vi "waveformTimeKeep.vi"(6 "DAQ Settings":T1={"RH/T Sensor VSS (V)"=5.048, "K0"=0.9054, "K1"=-2.995, "Offset"=0.0, "Gain"=1.0, "Samples/Channel/s"=1000.0, "Samples to Average"=100.0} {"Offset" step=0.01 format="%_3f"; "K1" format="%#_13g"; "K0" format="%#_13g"; "RH/T Sensor VSS (V)" format="%.3g"}, 8 "error in (no error)":errorcluster, 11 "input cluster":T2) -> (0 "error out":errorcluster, 2 "Samples/second":dbl, 3 "appended array":waveform(dbl)[](array[waveform]))   [LabVIEW 2020]
uses:
  typeDefs/Parameters.ctl
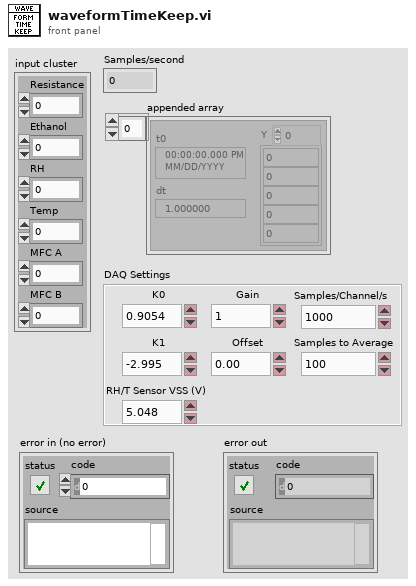
[diagram p1: front panel]
types:
  T1 = typedef "Parameters.ctl" = cluster{"RH/T Sensor VSS (V)":dbl, "K0":dbl, "K1":dbl, "Offset":dbl, "Gain":dbl, "Samples/Channel/s":dbl, "Samples to Average":dbl}
  T2 = cluster{"Resistance":dbl, "Ethanol":dbl, "RH":dbl, "Temp":dbl, "MFC A":dbl, "MFC B":dbl}
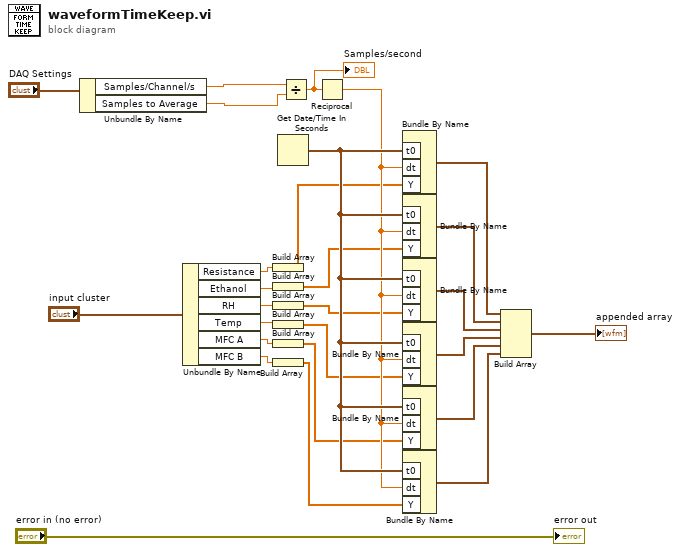
[diagram p0: block diagram]
diagram:
  n1 = Unbundle By Name("DAQ Settings") -> ("Samples/Channel/s"=w2:dbl, "Samples to Average"=w3:dbl)
  n2 = Unbundle By Name("input cluster") -> ("Resistance"=w24:dbl, "Ethanol"=w22:dbl, "RH"=w20:dbl, "Temp"=w18:dbl, "MFC A"=w16:dbl, "MFC B"=w14:dbl)
  n3 = Build Array(w24) -> (w23:dbl[])
  n4 = Build Array(w22) -> (w21:dbl[])
  n5 = Build Array(w20) -> (w19:dbl[])
  n6 = Build Array(w18) -> (w17:dbl[])
  n7 = Build Array(w16) -> (w15:dbl[])
  n8 = Build Array(w14) -> (w13:dbl[])
  n9 = Get Date/Time In Seconds() -> (seconds since 1Jan1904=w26:timestamp)
  n10 = Divide(x=w2, y=w3) -> (x/y=w1:dbl)
  "Samples/second" <- w1
  n11 = Reciprocal(x=w1) -> (1/x=w25:dbl)
  n12 = Bundle By Name("t0"=w26, "dt"=w25, "Y"=w23) -> (w12:waveform(dbl))  [unwired: 1 in]
  n13 = Bundle By Name("t0"=w26, "dt"=w25, "Y"=w21) -> (w11:waveform(dbl))  [unwired: 1 in]
  n14 = Bundle By Name("t0"=w26, "dt"=w25, "Y"=w19) -> (w10:waveform(dbl))  [unwired: 1 in]
  n15 = Bundle By Name("t0"=w26, "dt"=w25, "Y"=w17) -> (w9:waveform(dbl))  [unwired: 1 in]
  n16 = Bundle By Name("t0"=w26, "dt"=w25, "Y"=w15) -> (w8:waveform(dbl))  [unwired: 1 in]
  n17 = Bundle By Name("t0"=w26, "dt"=w25, "Y"=w13) -> (w7:waveform(dbl))  [unwired: 1 in]
  n18 = Build Array(w12, w11, w10, w9, w8, w7) -> (→"appended array":waveform(dbl)[])
  "error out" <- "error in (no error)"
